vi "Load.vi"(8 "error in (no error)":errorcluster, 10 "Path":path, 11 "Renderer":refnum<class "Renderer.lvclass">) -> (0 "error out":errorcluster, 3 "Animated Texture out":refnum<class "Animated Texture.lvclass">)   [LabVIEW 2015, in "Animated Texture.lvclass"]
uses:
  Animated Texture.lvclass
  Renderer/Renderer.lvclass
  Animated Texture.lvclass/Animated Texture.ctl
  Texture/Texture.lvclass
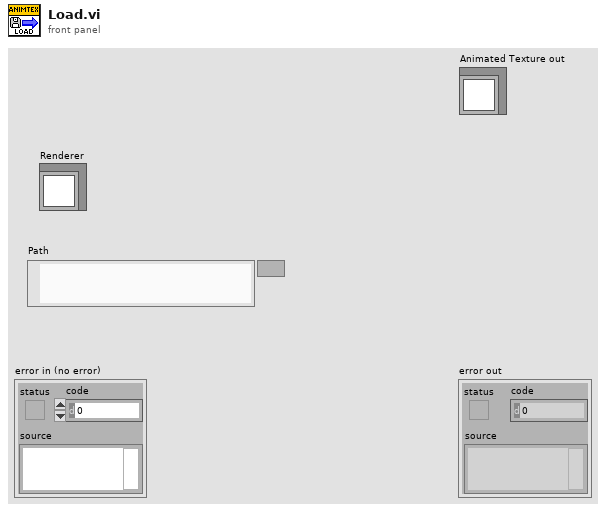
[diagram p1: front panel]
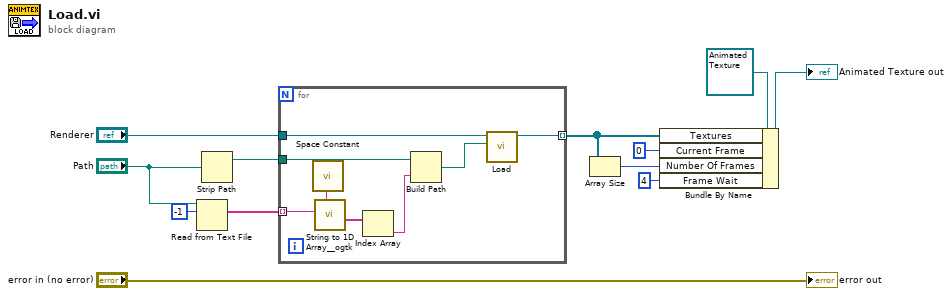
[diagram p0: block diagram]
diagram:
  n1 = Read from Text File(file (use dialog)="Path", count=-1) -> (text=w9:string[])  [unwired: 2 in, 3 out]
  n2 = Strip Path(path="Path") -> (stripped path=w7:path)  [unwired: 1 out]
  n3 = for {
    tunnel: "Renderer" -> [w14]
    tunnel: [w20] -> w4 mode=indexing
    tunnel: w9 -> [w18] mode=indexing
    tunnel: w7 -> [w19]
    n4 = call <vilib>:"Space Constant.vi"() -> ("String"=w17:string)
    n5 = call <userlib>:"String to 1D Array__ogtk.vi"("delimiter (Tab)"=w17, "string"=w18) -> ("Array of Strings"=w16:string[])  [unwired: 9 in]
    n6 = Index Array(array=w16) -> (element=w15:string)  [unwired: 1 in]
    n7 = Build Path(base path=w19, name or relative path=w15) -> (appended path=w13:path)
    n8 = call "Load.vi"("Path"=w13, "Renderer"=w14) -> ("Texture out"=w20:refnum<class "Texture.lvclass">)  [unwired: 9 in]
  }
  n9 = Array Size(array=w4) -> (size(s)=w3:i32)
  n10 = Bundle By Name(cluster=refnum<class "Animated Texture.lvclass"> refnum ("Animated Texture in"), "Textures"=w4, "Current Frame"=0, "Number Of Frames"=w3, "Frame Wait"=4) -> (→"Animated Texture out":refnum<class "Animated Texture.lvclass">)
  "error out" <- "error in (no error)"
